vi "Easy Grid Setup.vi"(6 "Images Path":path, 8 "error in":errorcluster, 9 "DataSource Data":string[][](array[string]), 10 "ColumnSetup":T1[](array[typedef]) {"MinWidth" min=2 step=1; "AutoSizeMode" items=["None"=1, "ColumnHeader"=2, "AllCellsExceptHeader"=4, "AllCells"=6, "DisplayedCellsExceptHeader"=8, "DisplayedCells"=10, "Fill"=16]; "FillWeight" min=1 max=100}, 11 "DataGridView":refnum<k24>) -> (0 "error out":errorcluster, 1 "registeredEvents":refnum<event-registration>, 2 "DataTable out":refnum<class "DataTable.lvclass">, 3 "DataGrid out":refnum<class "DataGridView.lvclass">)   [LabVIEW 2016, in "DataGrid.lvlib"]
doc: "Given a new datagridview .net container reference, this VI does all the sequencing and setup for your grid with a given input datasource table. It outputs the finished classes for datagrid and datatable, as well as the registered events for the grid that can be linked to an event structure for monitoring."
uses:
  <userlib>/LabVIEWdotNetDataGrid/source/DataGrid.lvlib
  <userlib>/LabVIEWdotNetDataGrid/source/Events/Abstract EVENT/Abstract EVENT.lvclass
  System.Windows.Forms
  <userlib>/LabVIEWdotNetDataGrid/source/GridColumn/ColumnDefinition.ctl
  <userlib>/LabVIEWdotNetDataGrid/source/GridColumn/ColumnType.ctl
  <userlib>/LabVIEWdotNetDataGrid/source/DataTable/DataTable.lvclass
  <userlib>/LabVIEWdotNetDataGrid/source/DataGridView/DataGridView.lvclass
  <userlib>/LabVIEWdotNetDataGrid/source/DataTable/Add Rows (String).vi
  <userlib>/LabVIEWdotNetDataGrid/source/GridColumn/GridColumn.lvclass
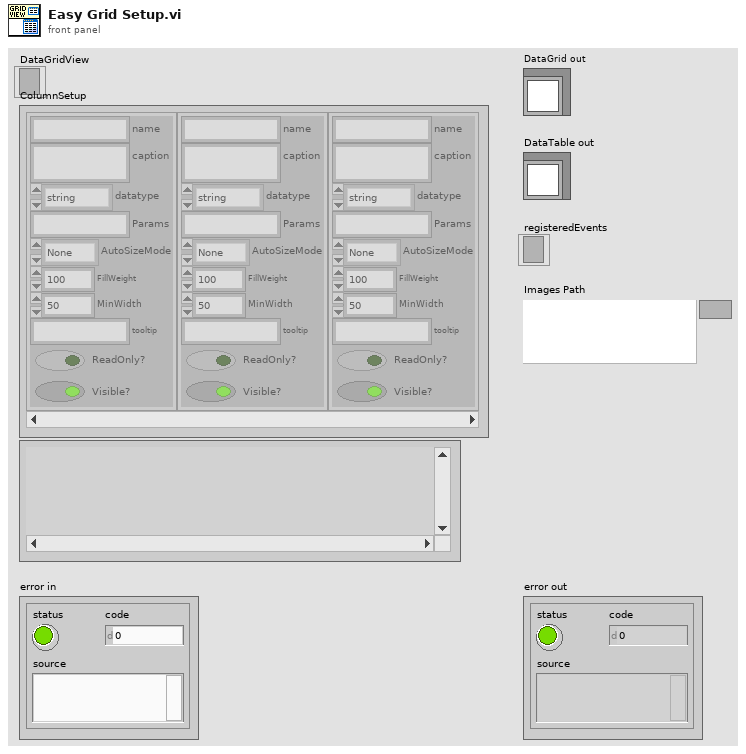
[diagram p1: front panel]
types:
  T1 = typedef "DataGrid.lvlib/GridColumn.lvclass/ColumnDefinition.ctl" = cluster{"name":string, "caption":string, "datatype":T2, "Params":string, "AutoSizeMode":i32, "FillWeight":sgl, "MinWidth":u32, "tooltip":string, "ReadOnly?":bool, "Visible?":bool}
  T2 = typedef "DataGrid.lvlib/GridColumn.lvclass/ColumnType.ctl" = enum16{"string", "image", "check", "numeric", "timestamp", "button", "combo", "link"}
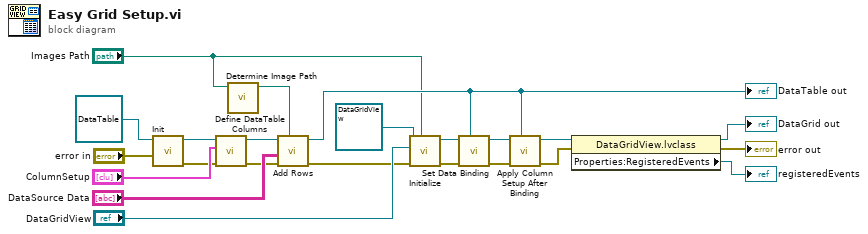
[diagram p0: block diagram]
diagram:
  n1 = call <userlib>:"Init.vi"("error in (no error)"="error in", "DataTable in"=refnum<class "DataTable.lvclass"> refnum) -> ("error out"=w17:errorcluster, "DataTable out"=w19:refnum<class "DataTable.lvclass">)  [unwired: 8 in]
  n2 = call <userlib>:"Define DataTable Columns.vi"("error in (no error)"=w17, "ColumnSetup"="ColumnSetup", "DataTable In"=w19) -> ("error out"=w15:errorcluster, "DataTable Out"=w18:refnum<class "DataTable.lvclass">)  [unwired: 7 in]
  n3 = call <userlib>:"Determine Image Path.vi"("image path"="Images Path") -> ("Path"=w1:path)  [unwired: 10 in]
  n4 = call-poly <userlib>:"Add Rows.vi"("image path"=w1, "error in (no error)"=w15, "String Data"="DataSource Data", "DataTable in"=w18) -> ("error out"=w11:errorcluster, "DataTable out"=w10:refnum<class "DataTable.lvclass">)  [unwired: 6 in]
  "DataTable out" <- w10
  n5 = call <userlib>:"Initialize.vi"("image path"="Images Path", "error in"=w11, "DataGridView"="DataGridView", "DataGrid in"=refnum<class "DataGridView.lvclass"> refnum) -> ("error out"=w12:errorcluster, "DataGrid out"=w13:refnum<class "DataGridView.lvclass">)  [unwired: 6 in]
  n6 = call <userlib>:"Set Data Binding.vi"("DataTable Source"=w10, "error in (no error)"=w12, "DataGridView in"=w13) -> ("error out"=w6:errorcluster, "DataGridView out"=w3:refnum<class "DataGridView.lvclass">)  [unwired: 7 in]
  n7 = call <userlib>:"Apply Column Setup After Binding.vi"("DataTable"=w10, "error in (no error)"=w6, "DataGridView in"=w3) -> ("error out"=w9:errorcluster, "DataGridView out"=w4:refnum<class "DataGridView.lvclass">)  [unwired: 7 in]
  n8 = property class="DataGridView.lvclass"(reference=w4, error in=w9) -> (reference out=→"DataGrid out":refnum<class "DataGridView.lvclass">, error out=→"error out":errorcluster, "Properties:RegisteredEvents"=→"registeredEvents":refnum<event-registration>)
